vi "ReverseDrive.vi"(7 "cReverseDrive":bool, 9 "Right":dbl, 10 "Left":dbl) -> (1 "Right":dbl, 2 "Left":dbl)   [LabVIEW 2013]
doc: "Reverses driving, back is driven as front would be in a forward drive."
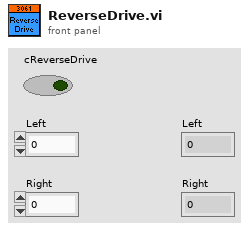
[diagram p1: front panel]
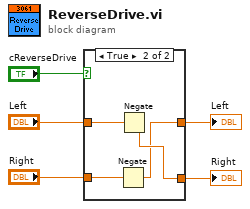
[diagram p0: block diagram]
diagram:
  n1 = case shown="True" "cReverseDrive" {
    tunnel: [w7 w8] -> w3
    tunnel: "Left" -> [w7 w10]
    tunnel: [w6 w9] -> w1
    tunnel: "Right" -> [w6 w11]
    frame False {
    }
    frame True {
      n2 = Negate(x=w11) -> (-x=w8:dbl)
      n3 = Negate(x=w10) -> (-x=w9:dbl)
    }
  }
  "Left" <- w3
  "Right" <- w1
